vi "Command prefix add.vi"(0 "Command_Types":T3, 1 "Status":T1, 5 "command":T2, 11 "error in (no error)":errorcluster) -> (6 "command str":string, 8 "prefix+cmd":string, 15 "error out":errorcluster)   [LabVIEW 2019, in "mmW_commands.lvlib"]
uses:
  mmW_commands.lvlib
  TypeDefs/command_types.ctl
  TypeDefs/commands.ctl
  TypeDefs/response status.ctl
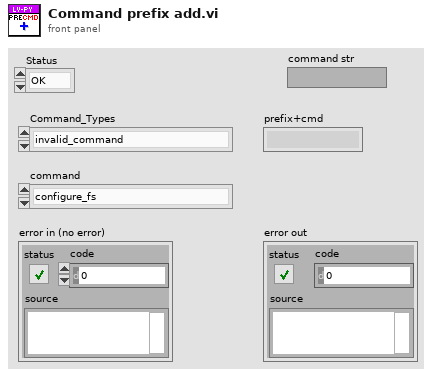
[diagram p1: front panel]
types:
  T1 = typedef "mmW_commands.lvlib/response status.ctl" = enum16{"OK", "Error", "Warning", "Unknown"}
  T2 = typedef "mmW_commands.lvlib/commands.ctl" = enum16{"configure_fs", "configure_rf", "configure_trigger", "equalization_enable", "equalization_start", "lo_sync_enable", "equalization_stop", "get_instrument_status", "get_versions", "initialize_hw", "pop_rx", "set_log_level", "Shutdown", "start", "start_instrument_app", "stop", "trans", "transceive", "trigger_burst", "trigger_sync_enable", "Write TX", "resp_generic", "resp_waveform", "send_trigger", "fetch", "transceive2"}
  T3 = typedef "mmW_commands.lvlib/command_types.ctl" = enum16{"invalid_command", "instrument_control", "environment_control", "response"}
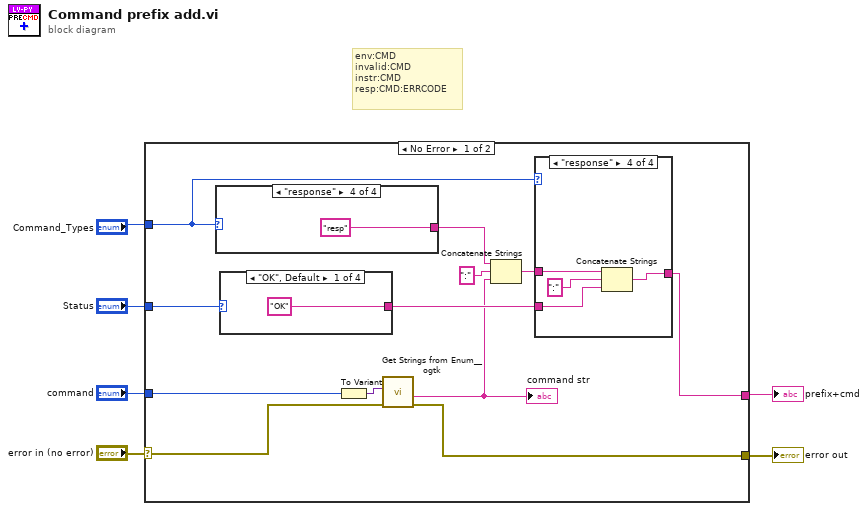
[diagram p0: block diagram]
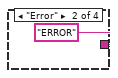
[diagram p5: hidden frame]
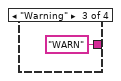
[diagram p6: hidden frame]
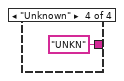
[diagram p7: hidden frame]
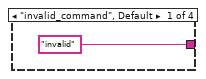
[diagram p8: hidden frame]
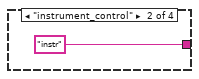
[diagram p9: hidden frame]
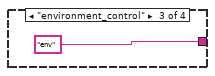
[diagram p10: hidden frame]
diagram:
  # "env:CMD\ninvalid:CMD\ninstr:CMD\nresp:CMD:ERRCODE"
  n1 = case shown="No Error" "error in (no error)" {
    selector: "error in (no error)" -> [w15 w34]
    tunnel: "command" -> [w17 _]
    tunnel: [w16 w34] -> w3
    tunnel: [w14 _] -> w4
    tunnel: "Command_Types" -> [w11 _]
    tunnel: "Status" -> [w13 _]
    frame No Error {
      n2 = case shown="\"response\"" w11 {
        tunnel: ["invalid" "instr" "env" "resp" ("string")] -> w9
        frame "invalid_command", Default {
        }
        frame "instrument_control" {
        }
        frame "environment_control" {
        }
        frame "response" {
        }
      }
      n3 = case shown="\"OK\", Default" w13 {
        tunnel: ["OK" ("string") "ERROR" ("string") "WARN" ("string") "UNKN" ("string")] -> w12
        frame "OK", Default {
        }
        frame "Error" {
        }
        frame "Warning" {
        }
        frame "Unknown" {
        }
      }
      n4 = To Variant(anything=w17) -> (Variant=w18:variant)
      n5 = call <userlib>:"Get Strings from Enum__ogtk.vi"("error in (no error)"=w15, "Enum"=w18) -> ("error out"=w16:errorcluster, "String Value"=w8:string)  [unwired: 6 in, 2 out]
      "command str" <- w8
      n6 = Concatenate Strings(w9, ":" ("string"), w8) -> (w7:string)
      n7 = case shown="\"response\"" w11 {
        tunnel: [w19 w20 w21 w25] -> w14
        tunnel: w12 -> [_ _ _ w22]
        tunnel: w7 -> [w19 w20 w21 w23]
        frame "invalid_command", Default {
        }
        frame "instrument_control" {
        }
        frame "environment_control" {
        }
        frame "response" {
          n8 = Concatenate Strings(w23, ":" ("string"), w22) -> (w25:string)
        }
      }
    }
    frame Error {
    }
  }
  "prefix+cmd" <- w4
  "error out" <- w3
